vi "Controller Report Error.vi"(8 "error in":errorcluster, 10 "Error location":string) -> (0 "error out":errorcluster)   [LabVIEW 2011, in "Controller VIs.lvlib"]
uses:
  Controller VIs.lvlib
  <vilib>/NI_Real-Time Target Support.lvlib
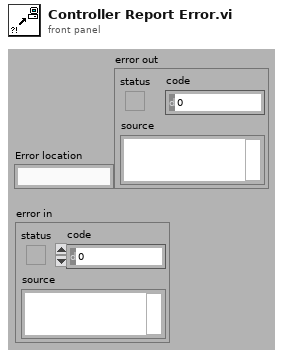
[diagram p1: front panel]
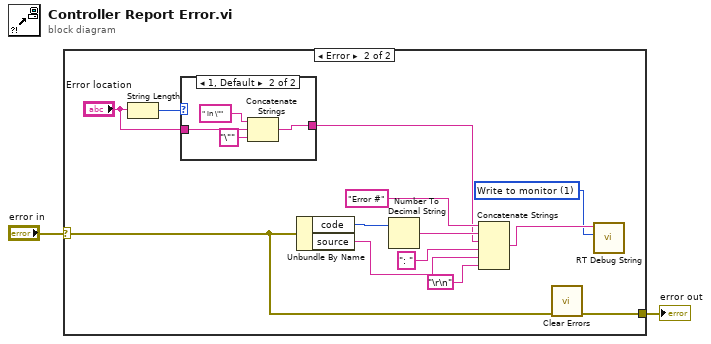
[diagram p0: block diagram]
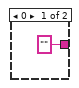
[diagram p3: hidden frame]
diagram:
  n1 = case shown="Error" "error in" {
    selector: "error in" -> [w3 w4]
    tunnel: [w3 w5] -> w1
    frame No Error {
    }
    frame Error {
      w12 = u16 1 items=["Write to serial", "Write to monitor"] ("Interface")
      n2 = String Length(string="Error location") -> (length=w11:i32)
      n3 = case shown="1, Default" w11 {
        tunnel: "Error location" -> [_ w20]
        tunnel: ["" w19] -> w7
        frame 0 {
        }
        frame 1, Default {
          n4 = Concatenate Strings(" in \"" ("string"), w20, "\"" ("string")) -> (w19:string)
        }
      }
      n5 = Unbundle By Name(w4) -> ("code"=w16:i32, "source"=w9:string)
      n6 = Number To Decimal String(number=w16) -> (decimal integer string=w14:string)  [unwired: 1 in]
      n7 = Concatenate Strings("Error #", w14, w7, ": ", w9, "\r\n") -> (w13:string)
      n8 = call <vilib>:"Clear Errors.vi"("error in (no error)"=w4) -> ("error out"=w5:errorcluster)  [unwired: 6 in]
      n9 = call <vilib>:"RT Debug String.vi"("Interface"=w12, "String to write"=w13) -> ()  [unwired: 9 in, 1 out]
    }
  }
  "error out" <- w1
